vi "Add row item.vi"(10 "SP P":dbl, 11 "Data Cluster in":T1 {"Pump_data"."mix rpm" format="%.2f"; "Pump_data"."Volume corrected" format="%.2f"; "Pump_data"."Position_MM" format="%.3f"; "Pump_data"."Volume PV" format="%.2f"; "Pump_data"."Flow PV" format="%#.6f"; "Pump_data"."Pressure PV" format="%.3f"}) -> (0 "error out":errorcluster, 3 "Data Cluster out":T1 {"Pump_data"."mix rpm" format="%.2f"; "Pump_data"."Volume corrected" format="%.2f"; "Pump_data"."Position_MM" format="%.3f"; "Pump_data"."Volume PV" format="%.2f"; "Pump_data"."Flow PV" format="%#.6f"; "Pump_data"."Pressure PV" format="%.3f"})   [LabVIEW 2023, in "AutoPV.lvlib"]
uses:
  AutoPV.lvlib
  Module Data--cluster.ctl
  <vilib>/ActorFramework/Message Enqueuer/Message Enqueuer.lvclass
  Drive/Pump_Data_Type.ctl
  Initial Data/InitalData Type.ctl
  Drive/Drive.lvlib
  Initial Data/Initial Data.lvlib
panel:
  # "Образец"
  # "Образец"
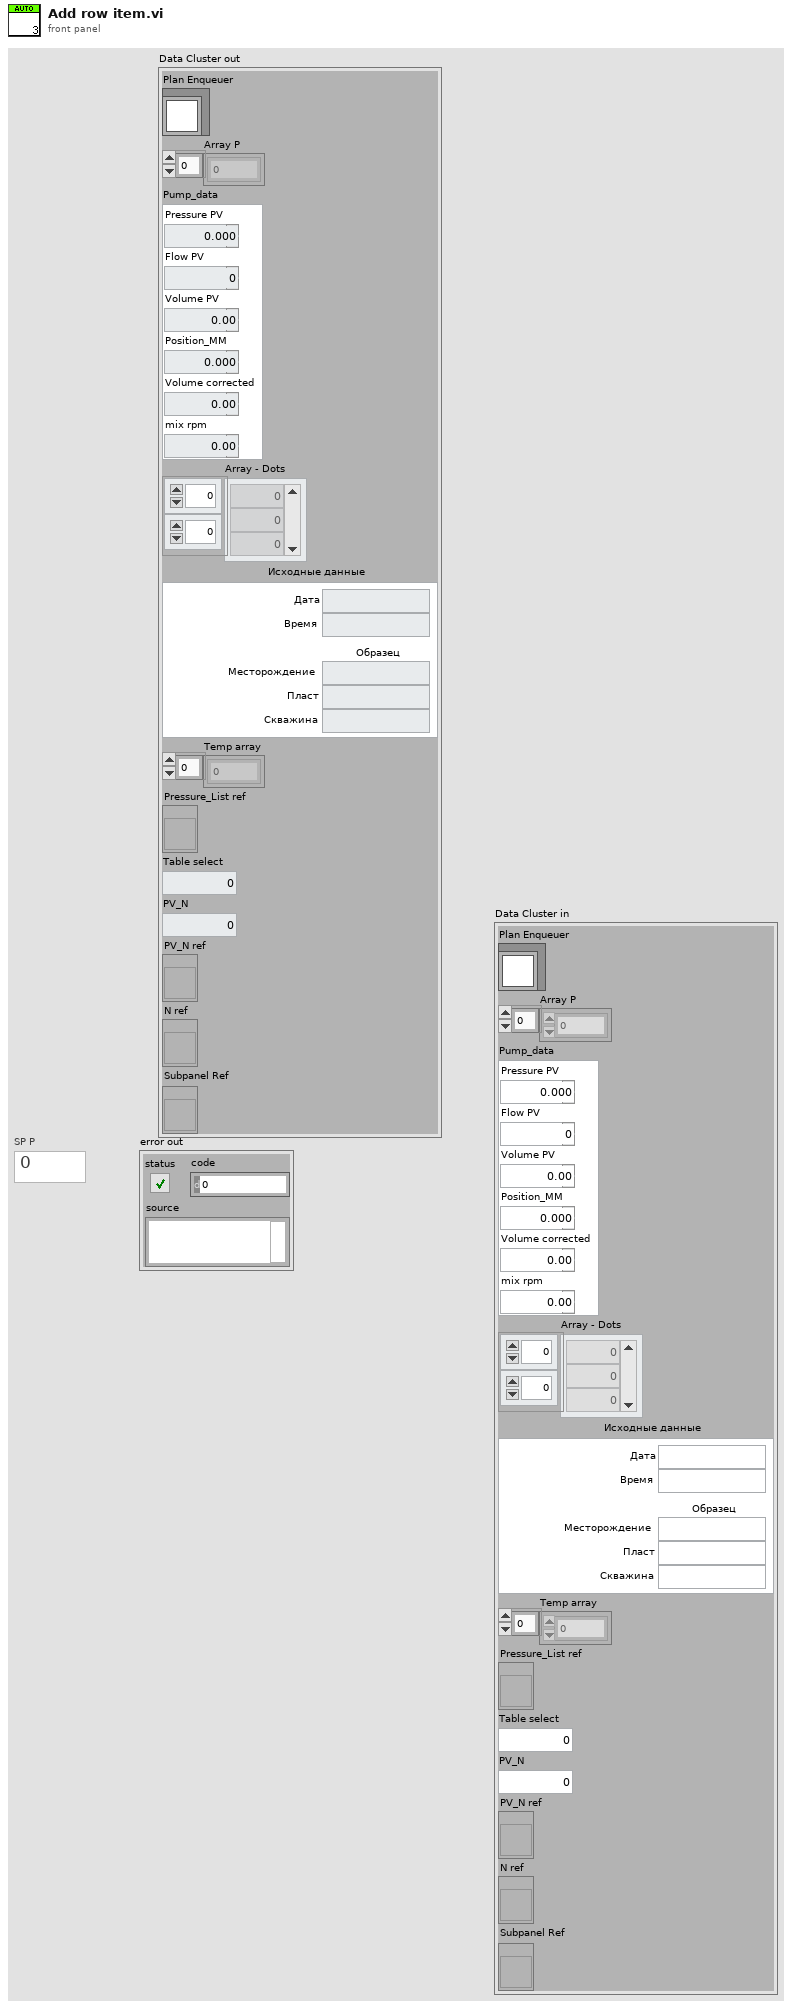
[diagram p1: front panel]
types:
  T1 = typedef "AutoPV.lvlib/Module Data--cluster.ctl" = cluster{"Plan Enqueuer":refnum<class "Message Enqueuer.lvclass">, "Array P":dbl[], "Pump_data":T2, "Array - Dots":dbl[][], "Исходные данные":T3, "Temp array":dbl[], "Pressure_List ref":refnum<vi>, "Table select":i32, "PV_N":i32, "PV_N ref":refnum<vi>, "N ref":refnum<vi>, "Subpanel Ref":refnum<vi>}
  T2 = typedef "Drive.lvlib/Pump_Data_Type.ctl" = cluster{"Pressure PV":dbl, "Flow PV":dbl, "Volume PV":dbl, "Position_MM":dbl, "Volume corrected":dbl, "mix rpm":dbl}
  T3 = typedef "Initial Data.lvlib/InitalData Type.ctl" = cluster{"Дата":string, "Время":string, "Месторождение":string, "Пласт":string, "Скважина":string}
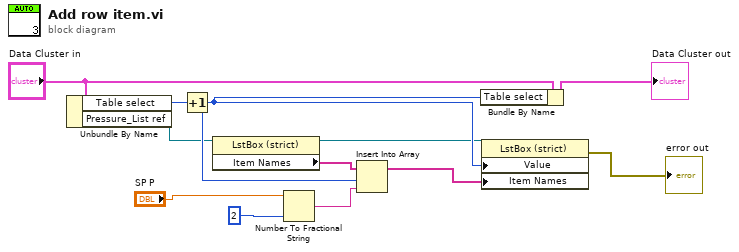
[diagram p0: block diagram]
diagram:
  n1 = Unbundle By Name("Data Cluster in") -> ("Table select"=w10:i32, "Pressure_List ref"=w3:refnum<vi>)
  n2 = Increment(x=w10) -> (x+1=w12:i32)
  n3 = property class="LstBox (strict)"(reference=w3) -> (reference out=w5:refnum<vi>, "Item Names"=w6:string[])  [unwired: 1 in, 1 out]
  n4 = Number To Fractional String(number="SP P", precision (6)=i16 2) -> (F-format string=w7:string)  [unwired: 2 in]
  n5 = Insert Into Array(array=w6, index=w12, new element=w7) -> (w8:string[])
  n6 = Bundle By Name(cluster="Data Cluster in", "Table select"=w12) -> (→"Data Cluster out":T1)
  n7 = property class="LstBox (strict)"(reference=w5, "Value"=w12, "Item Names"=w8) -> (error out=→"error out":errorcluster)  [unwired: 1 in, 1 out]
